vi "get Image Description.vi"(8 "error in":errorcluster, 10 "imageID":u32, 11 "cycloneHandle":u32) -> (0 "error out":errorcluster, 3 "function return":string)   [LabVIEW 2021, in "CycloneControlSDK.lvlib"]
doc: "extern \"C\" char * _cdecl getImageDescription(uint32_t cycloneHandle, uint32_t imageID);"
uses:
  CycloneControlSDK.lvlib
  CycloneControlSDK_64.dll
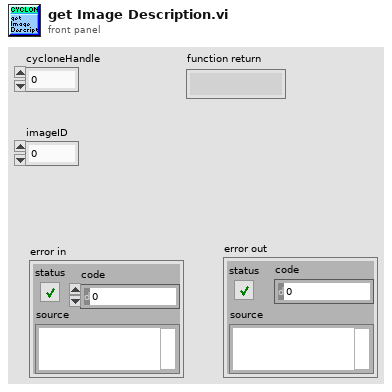
[diagram p1: front panel]
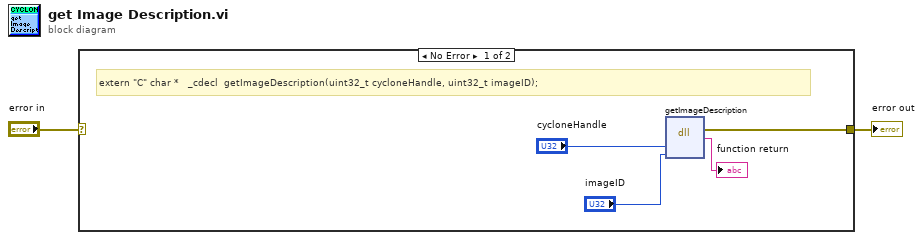
[diagram p0: block diagram]
diagram:
  n1 = case shown="No Error" "error in" {
    selector: "error in" -> [_ w7]
    tunnel: [w3 w7] -> w1
    frame No Error {
      # "extern \"C\" char *   _cdecl  getImageDescription(uint32_t cycloneHandle, uint32_t imageID);"
      n2 = dll-call lib="C:/PEMicro/cyclone/cycloneControl/controlsdk/examples/labview2018/user.lib/CycloneControlSDK/CycloneControlSDK_64.dll" fn="getImageDescription"("cycloneHandle"="cycloneHandle", "imageID"="imageID") -> (error out=w3:errorcluster, "return type"=→"function return":string)  [unwired: 5 in, 1 out]
    }
    frame Error {
    }
  }
  "error out" <- w1
